vi "loadPCDispatch.vi"(10 "template (empty)":path=path "C:/Users/yy/Downloads/機台排程-(0611)MPS後修改2200.xls") -> (0 "error out 2":errorcluster)   [LabVIEW 2012]
uses:
  <vilib>/Utility/NIReport.llb/NI_report.lvclass
  <vilib>/addons/database/Connection.llb/DB Tools Open Connec (Path).vi
  <vilib>/addons/database/Connection.llb/Conn Execute.vi
  <vilib>/addons/database/Recordset.llb/Rec Destroy - Connection.vi
  <vilib>/addons/_office/excel.llb/Excel Get Data (str).vi
  <vilib>/Utility/NIReport.llb/Excel/NI_Excel.lvclass
  <vilib>/addons/_office/NI_ReportGenerationToolkit.lvlib
  <vilib>/addons/database/NI_Database_API.lvlib
panel:
  out "data":string
  out "x .and. y?":bool
  out "error out 4":errorcluster
  out "array":string[][](array[string])
  out "substring":string
  in  "start (0, 0)":cluster{"start row":i32, "start column":i32}
  out "row":i32
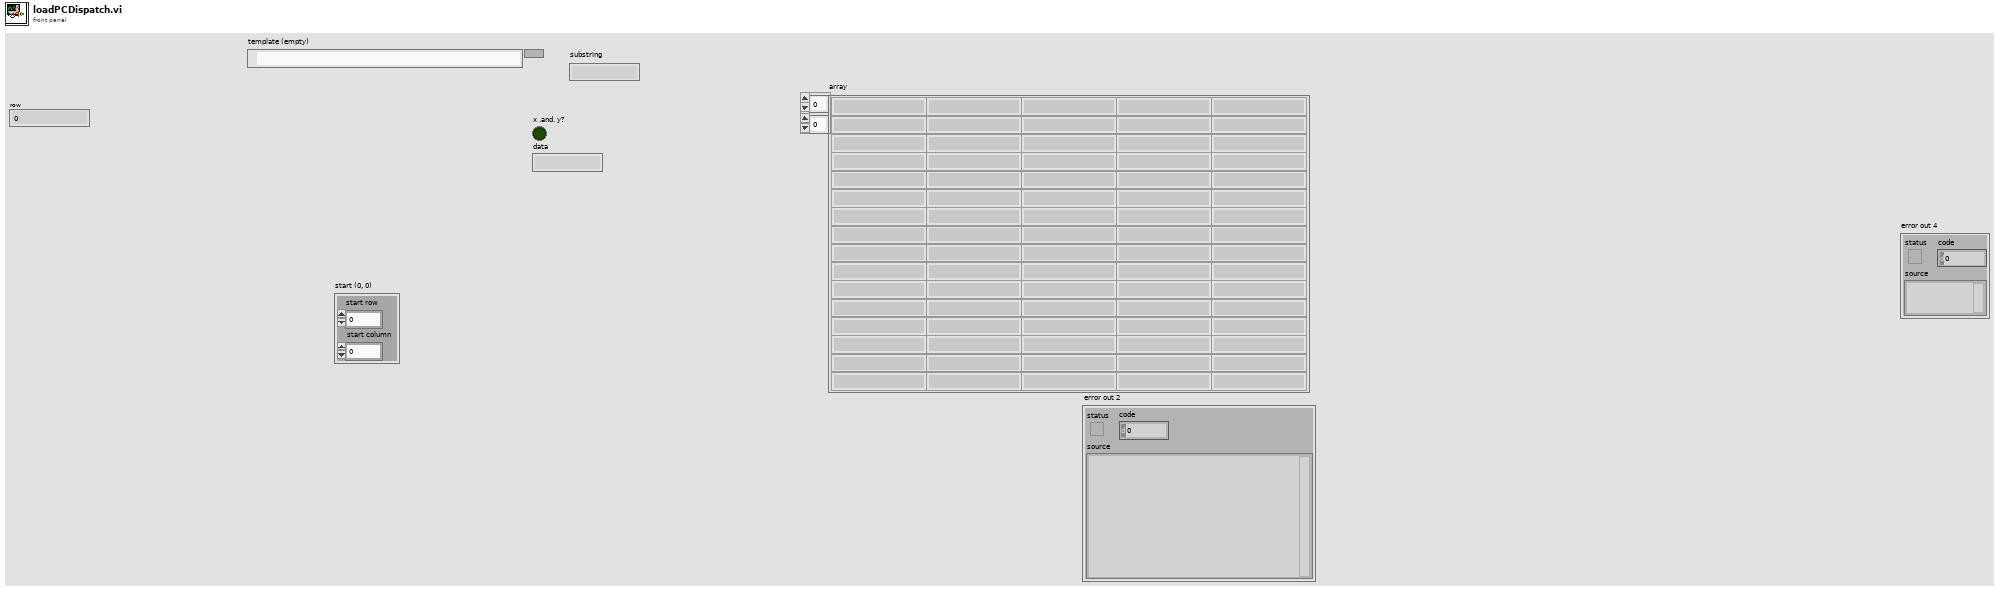
[diagram p1: front panel]
types:
  T1 = enum16{"Standard Report", "HTML", "Word", "Excel"}
  T2 = typedef "NI_Database_API.lvlib/Conn ObjectReference.ctl" = refnum<k1>
  T3 = typedef "NI_Database_API.lvlib/Rec ObjectReference.ctl" = refnum<k1>
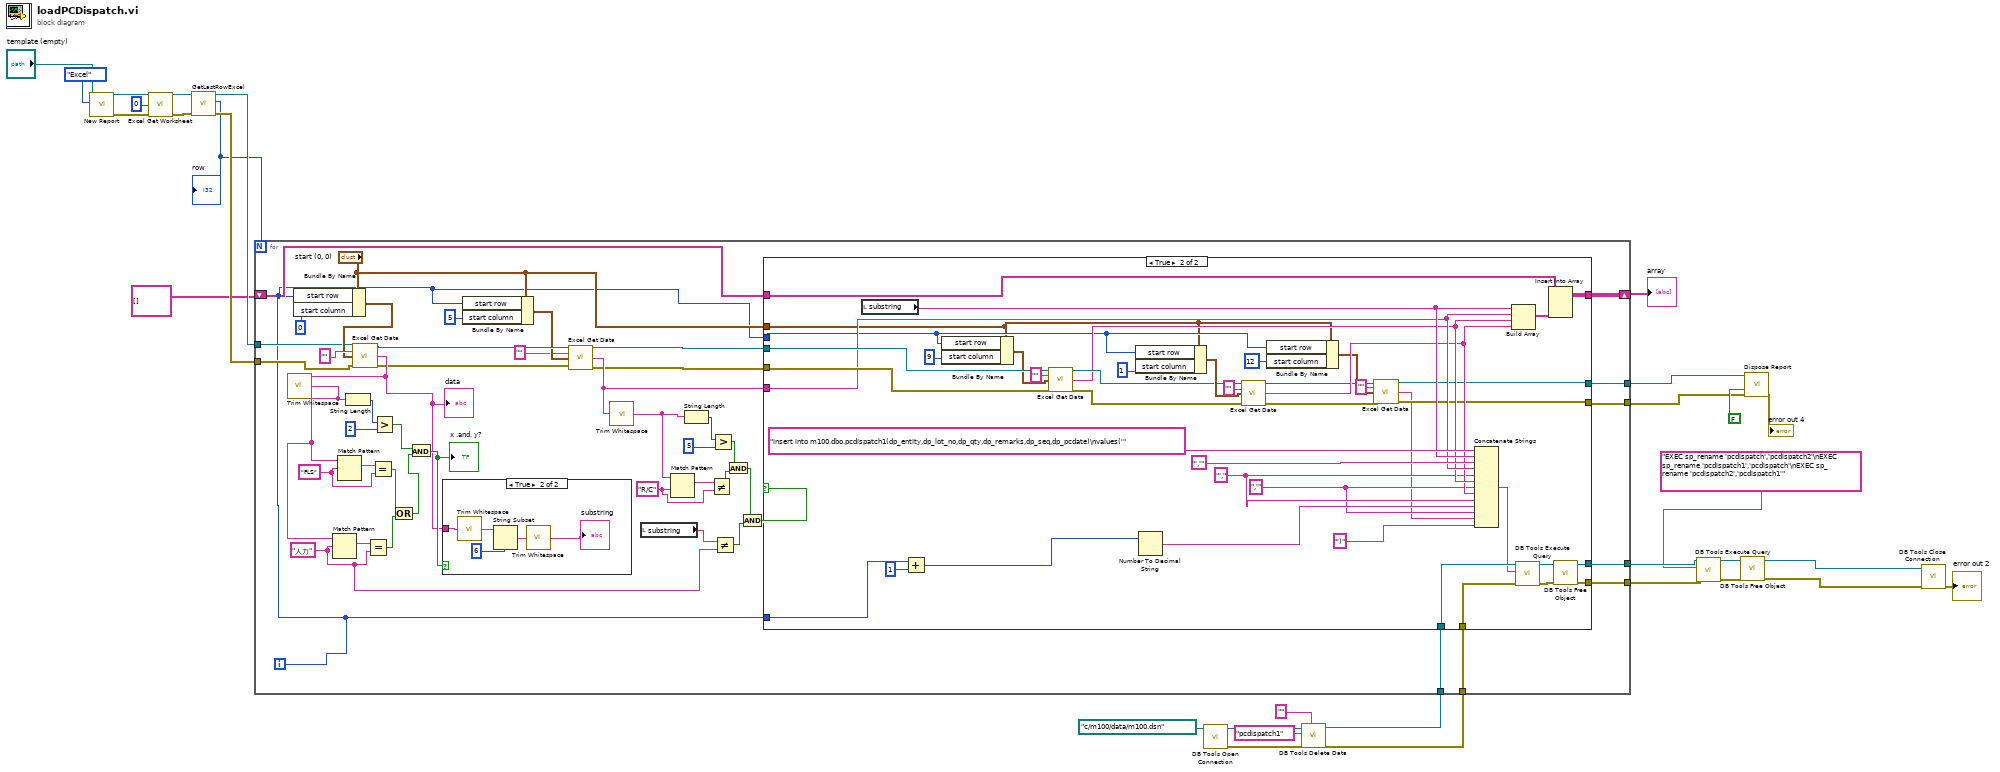
[diagram p0: block diagram]
diagram:
  n1 = call <vilib>:"New Report.vi"("report type"=T1."Excel" ("Report Type"), "template (empty)"="template (empty)") -> ("report out"=w30:refnum<class "NI_report.lvclass">, "error out"=w29:errorcluster)  [unwired: 12 in]
  n2 = call <vilib>:"Excel Get Worksheet.vi"("report in"=w30, "worksheet index (0)"=0, "error in (no error)"=w29) -> ("report out"=w28:refnum<class "NI_report.lvclass">, "error out"=w27:errorcluster)  [unwired: 11 in]
  n3 = call "GetLastRowExcel.vi"("error in (no error)"=w27, "report in"=w28) -> ("error out"=w24:errorcluster, "row"=w1:i32, "report out"=w23:refnum<class "NI_report.lvclass">)  [unwired: 7 in]
  "row" <- w1
  n4 = call-poly <vilib>:"DB Tools Open Connection.vi"("connection information"=path "c:/m100/data/m100.dsn") -> ("error out"=w17:errorcluster, "connection reference"=w18:T2)  [unwired: 7 in]
  n5 = call <vilib>:"DB Tools Delete Data.vi"("condition"="", "error in (no error)"=w17, "table"="pcdispatch1", "connection reference"=w18) -> ("error out"=w15:errorcluster, "connection reference out"=w16:T2)  [unwired: 6 in]
  n6 = for {
    N: w1 -> [_]
    tunnel: w23 -> [w73]
    tunnel: w24 -> [w72]
    shift-right: [w54] -> w21
    shift-left: string[][] [] ("array") -> [w53]
    tunnel: w16 -> [w48]
    tunnel: w15 -> [w45]
    tunnel: [w47] -> w6
    tunnel: [w46] -> w5
    tunnel: [w44] -> w10
    tunnel: [w43] -> w9
    i -> [w32]
    w36 = "人力" ("regular expression")
    w52 = "R/C" ("regular expression")
    w70 = "FLS" ("regular expression")
    n7 = Bundle By Name(cluster="start (0, 0)", "start row"=w32, "start column"=0) -> (w74:cluster{"start row":i32, "start column":i32})
    n8 = call-poly <vilib>:"Excel Get Data.vi"("report in"=w73, "data type"="", "start (0, 0)"=w74, "error in (no error)"=w72) -> ("report out"=w66:refnum<class "NI_report.lvclass">, "data"=w67:string, "error out"=w65:errorcluster)  [unwired: 9 in]
    "data" <- w67
    n9 = call <vilib>:"Trim Whitespace.vi"("string"=w67) -> ("trimmed string"=w42:string)  [unwired: 1 in]
    n10 = Match Pattern(string=w42, regular expression=w36) -> (match substring=w41:string)  [unwired: 1 in, 3 out]
    n11 = Match Pattern(string=w42, regular expression=w70) -> (match substring=w71:string)  [unwired: 1 in, 3 out]
    n12 = String Length(string=w42) -> (length=w75:i32)
    n13 = Equal?(x=w41, y=w36) -> (x = y?=w39:bool)
    n14 = Equal?(x=w71, y=w70) -> (x = y?=w40:bool)
    n15 = Greater?(x=w75, y=2) -> (0:w69:bool)
    n16 = Or(x=w40, y=w39) -> (x .or. y?=w38:bool)
    n17 = And(x=w69, y=w38) -> (x .and. y?=w68:bool)
    "x .and. y?" <- w68
    n18 = case shown="True" w68 {
      tunnel: w67 -> [_ w130]
      frame False {
      }
      frame True {
        n19 = call <vilib>:"Trim Whitespace.vi"("string"=w130) -> ("trimmed string"=w129:string)  [unwired: 1 in]
        n20 = String Subset(string=w129, length (rest)=6 ("length (rest)")) -> (substring=w128:string)  [unwired: 1 in]
        n21 = call <vilib>:"Trim Whitespace.vi"("string"=w128) -> ("trimmed string"=→"substring":string)  [unwired: 1 in]
      }
    }
    n22 = Bundle By Name(cluster="start (0, 0)", "start row"=w32, "start column"=5) -> (w63:cluster{"start row":i32, "start column":i32})
    n23 = call-poly <vilib>:"Excel Get Data.vi"("report in"=w66, "data type"="", "start (0, 0)"=w63, "error in (no error)"=w65) -> ("report out"=w51:refnum<class "NI_report.lvclass">, "data"=w55:string, "error out"=w50:errorcluster)  [unwired: 9 in]
    n24 = call <vilib>:"Trim Whitespace.vi"("string"=w55) -> ("trimmed string"=w59:string)  [unwired: 1 in]
    n25 = local read "substring"() -> (w37:string)
    n26 = Match Pattern(string=w59, regular expression=w52) -> (match substring=w58:string)  [unwired: 1 in, 3 out]
    n27 = String Length(string=w59) -> (length=w60:i32)
    n28 = Not Equal?(x=w58, y=w52) -> (x != y?=w57:bool)
    n29 = Greater?(x=w60, y=5) -> (0:w56:bool)
    n30 = Not Equal?(x=w37, y=w36) -> (x != y?=w35:bool)
    n31 = And(x=w56, y=w57) -> (x .and. y?=w34:bool)
    n32 = And(x=w34, y=w35) -> (x .and. y?=w33:bool)
    n33 = case shown="True" w33 {
      tunnel: w55 -> [_ w110]
      tunnel: [w83 w125] -> w54
      tunnel: w53 -> [w83 w124]
      tunnel: w51 -> [w80 w123]
      tunnel: w50 -> [w79 w122]
      tunnel: "start (0, 0)" -> [_ w89]
      tunnel: w32 -> [_ w91]
      tunnel: w48 -> [w82 w107]
      tunnel: [w82 w102] -> w47
      tunnel: [w81 w101] -> w46
      tunnel: w45 -> [w81 w106]
      tunnel: [w80 w93] -> w44
      tunnel: [w79 w92] -> w43
      tunnel: w32 -> [_ w97]
      frame False {
      }
      frame True {
        w86 = ",'" ("string")
        w99 = "'," ("string")
        n34 = local read "substring"() -> (w112:string)
        n35 = Add(x=w97, y=1) -> (x+y=w96:i32)
        n36 = Bundle By Name(cluster=w89, "start row"=w91, "start column"=9) -> (w120:cluster{"start row":i32, "start column":i32})
        n37 = call-poly <vilib>:"Excel Get Data.vi"("report in"=w123, "data type"="", "start (0, 0)"=w120, "error in (no error)"=w122) -> ("report out"=w115:refnum<class "NI_report.lvclass">, "data"=w109:string, "error out"=w114:errorcluster)  [unwired: 9 in]
        n38 = Bundle By Name(cluster=w89, "start row"=w91, "start column"=1) -> (w117:cluster{"start row":i32, "start column":i32})
        n39 = Number To Decimal String(number=w96) -> (decimal integer string=w100:string)  [unwired: 1 in]
        n40 = call-poly <vilib>:"Excel Get Data.vi"("report in"=w115, "data type"="", "start (0, 0)"=w117, "error in (no error)"=w114) -> ("report out"=w95:refnum<class "NI_report.lvclass">, "data"=w108:string, "error out"=w94:errorcluster)  [unwired: 9 in]
        n41 = Bundle By Name(cluster=w89, "start row"=w91, "start column"=12) -> (w88:cluster{"start row":i32, "start column":i32})
        n42 = call-poly <vilib>:"Excel Get Data.vi"("report in"=w95, "data type"="", "start (0, 0)"=w88, "error in (no error)"=w94) -> ("report out"=w93:refnum<class "NI_report.lvclass">, "data"=w85:string, "error out"=w92:errorcluster)  [unwired: 9 in]
        n43 = Concatenate Strings("insert into m100.dbo.pcdispatch1(dp_entity,dp_lot_no,dp_qty,dp_remarks,dp_seq,dp_pcdate)\nvalues('" ("string"), w112, "','" ("string"), w110, w99, w109, w86, w108, w99, w100, w86, w85, "')" ("string")) -> (w105:string)
        n44 = Build Array(w112, w110, w109, w108) -> (w126:string[])
        n45 = call-poly <vilib>:"DB Tools Execute Query.vi"("error in (no error)"=w106, "SQL query"=w105, "connection reference"=w107) -> ("error out"=w103:errorcluster, "recordset reference"=w104:T3)  [unwired: 5 in]
        n46 = Insert Into Array(array=w124, new element=w126) -> (w125:string[][])  [unwired: 2 in]
        n47 = call-poly <vilib>:"DB Tools Free Object.vi"("error in (no error)"=w103, "recordset reference"=w104) -> ("error out"=w101:errorcluster, "connection reference"=w102:T2)  [unwired: 8 in]
      }
    }
  }
  "array" <- w21
  n48 = call-poly <vilib>:"DB Tools Execute Query.vi"("error in (no error)"=w5, "SQL query"="EXEC sp_rename 'pcdispatch','pcdispatch2'\nEXEC sp_rename 'pcdispatch1','pcdispatch'\nEXEC sp_rename 'pcdispatch2','pcdispatch1'", "connection reference"=w6) -> ("error out"=w8:errorcluster, "recordset reference"=w7:T3)  [unwired: 5 in]
  n49 = call-poly <vilib>:"DB Tools Free Object.vi"("error in (no error)"=w8, "recordset reference"=w7) -> ("error out"=w3:errorcluster, "connection reference"=w4:T2)  [unwired: 8 in]
  n50 = call-dynamic "Dispose Report.vi"("report in"=w10, "save changes? (F)"=FALSE, "error in (no error)"=w9) -> ("error out"=→"error out 4":errorcluster)  [unwired: 12 in]
  n51 = call <vilib>:"DB Tools Close Connection.vi"("error in (no error)"=w3, "connection reference"=w4) -> ("error out"=→"error out 2":errorcluster)  [unwired: 5 in]
